vi "toplevel.vi"() -> ()   [LabVIEW 2017]
uses:
  <vilib>/Instr/_visa.llb/VISA Configure Serial Port (Instr).vi
  SPELS test.lvlib
panel:
  in  "путь до файл с отчётом":path=path "C:/Users/andreika/Documents/work/SPELS_TEST/stm_test/TestReport.xlsx"
  out "ЕСТЬ НЕПРОВЕРЕННЫЕ ДАННЫЕ":bool
  in  "считать массив":bool
  in  "загрузить массив":bool
  out "error out":errorcluster
  in  "перезапись/конкатенация":bool=TRUE
  in  "VISA resource name":refnum<visa-resource-name>
  in  "refresh array":bool=TRUE
  in  "stop":bool
  in  "файл с тестовым массивом":path
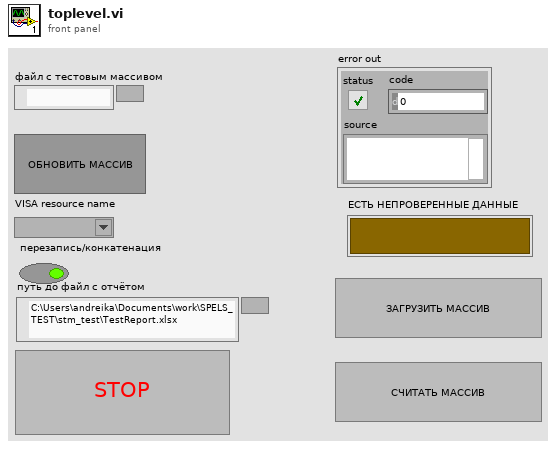
[diagram p1: front panel]
types:
  T1 = cluster{"elements 1 ":u8[], "elements 2":u8[], "bit numbers":string[], "single errors":u8, "double errors":u8}
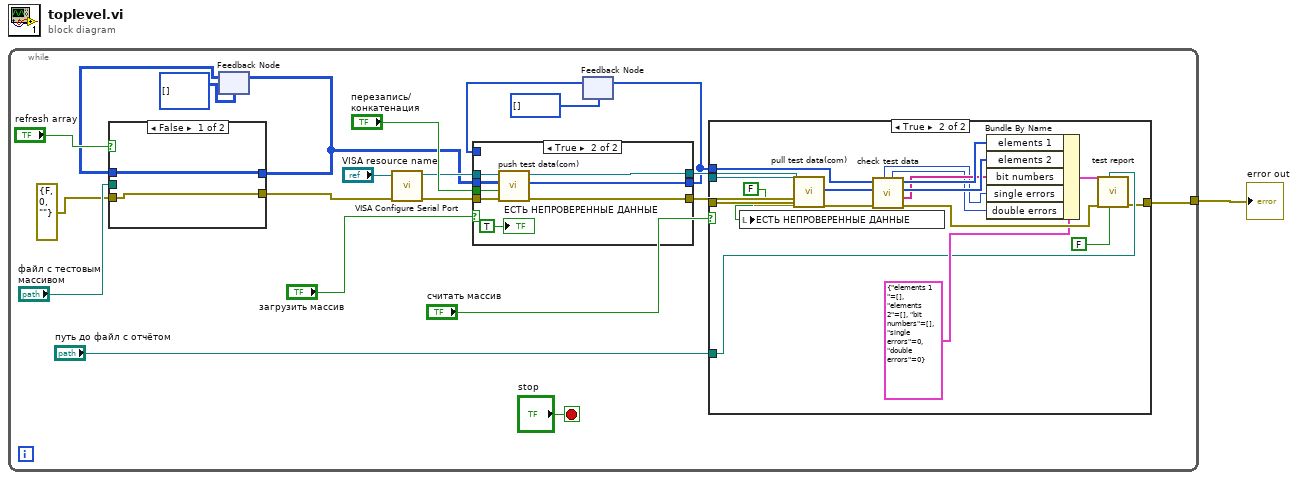
[diagram p0: block diagram]
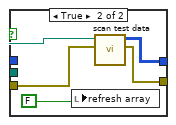
[diagram p4: hidden frame]
diagram:
  n1 = while {
    tunnel: [w4] -> w1
    stop <- "stop" stop-if-true
    n2 = feedback #1(u8[][] [] ("Array")) -> (w19:u8[][])
    n3 = case shown="False" "refresh array" {
      tunnel: [w53 w58] -> w11
      tunnel: "файл с тестовым массивом" -> [_ w57]
      tunnel: w19 -> [w53 _]
      tunnel: [w52 w55] -> w16
      tunnel: errorcluster {"status"=FALSE, "code"=0, "source"=""} ("error in") -> [w52 w54]
      frame False {
      }
      frame True {
        n4 = local write "refresh array"(FALSE ("refresh array")) -> ()
        n5 = call "scan test data.vi"("error in"=w54, "file path in"=w57) -> ("error out"=w55:errorcluster, "Array"=w58:u8[][])  [unwired: 7 in, 1 out]
      }
    }
    n6 = feedback-in #1(w11) -> ()
    n7 = call-poly "VISA Configure Serial Port"("VISA resource name"="VISA resource name", "error in (no error)"=w16) -> ("VISA resource name out"=w12:refnum<visa-resource-name>, "error out"=w14:errorcluster)  [unwired: 12 in]
    n8 = feedback #2(u8[] [] ("transmitted array")) -> (w9:u8[])
    n9 = case shown="True" "загрузить массив" {
      tunnel: w14 -> [w41 w51]
      tunnel: "перезапись/конкатенация" -> [_ w50]
      tunnel: w12 -> [w43 w49]
      tunnel: w11 -> [_ w48]
      tunnel: [w43 w47] -> w6
      tunnel: [w42 w46] -> w3
      tunnel: [w41 w45] -> w7
      tunnel: w9 -> [w42 _]
      frame False {
      }
      frame True {
        n10 = call "push test data(com).vi"("error in"=w51, "rewrite/concatenate"=w50, "array in"=w48, "VISA resource name in"=w49) -> ("error out"=w45:errorcluster, "transmitted array"=w46:u8[], "VISA resource name out"=w47:refnum<visa-resource-name>)  [unwired: 4 in, 1 out]
        "ЕСТЬ НЕПРОВЕРЕННЫЕ ДАННЫЕ" <- TRUE ("ЕСТЬ НЕПРОВЕРЕННЫЕ ДАННЫЕ")
      }
    }
    n11 = feedback-in #2(w3) -> ()
    n12 = case shown="True" "считать массив" {
      tunnel: w7 -> [w23 w40]
      tunnel: w6 -> [_ w39]
      tunnel: [w23 w24] -> w4
      tunnel: w3 -> [_ w37]
      tunnel: "путь до файл с отчётом" -> [_ w26]
      frame False {
      }
      frame True {
        n13 = local write "ЕСТЬ НЕПРОВЕРЕННЫЕ ДАННЫЕ"(FALSE) -> ()
        n14 = call "pull test data(com).vi"("error in"=w40, "VISA resource name in"=w39) -> ("error out"=w35:errorcluster, "received array"=w36:u8[])  [unwired: 7 in, 1 out]
        n15 = call "check test data.vi"("error in"=w35, "Array 2"=w36, "Array 1"=w37) -> ("error out"=w34:errorcluster, "bit numbers"=w29:string[], "elements 2"=w30:u8[], "elements 1"=w31:u8[], "double errors"=w28:i8, "single errors"=w27:i8)  [unwired: 2 in, 1 out]
        n16 = Bundle By Name(cluster=T1 {"elements 1 "=[], "elements 2"=[], "bit numbers"=[], "single errors"=0, "double errors"=0} ("test data cluster"), "elements 1"=w31, "elements 2"=w30, "bit numbers"=w29, "single errors"=w27, "double errors"=w28) -> (w32:T1)
        n17 = call "test report.vi"("append report?"=FALSE, "report path"=w26, "error in"=w34, "test data cluster"=w32) -> ("error out"=w24:errorcluster)  [unwired: 5 in, 2 out]
      }
    }
  }
  "error out" <- w1
